vi "AMZ_S3_AUTH_Create Date Header String in UTC.vi"(8 "error in (no error)":errorcluster) -> (0 "error out":errorcluster, 3 "DateTime String (UTC)":string)   [LabVIEW 2015, in "LV Interface for Amazon S3.lvlib"]
doc: "Create the DateTime string in the format Amazon needs. This string is necessary for every request as the Date header's value."
uses:
  LV Interface for Amazon S3.lvlib
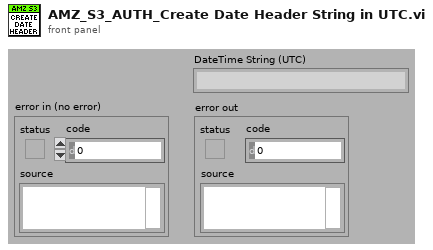
[diagram p1: front panel]
types:
  T1 = typedef "LVDateTimeRec.ctl" = cluster{"fractional second":dbl, "second":i32, "minute":i32, "hour":i32, "day of month":i32, "month":i32, "year":i32, "day of week":i32, "day of year":i32, "DST":i32}
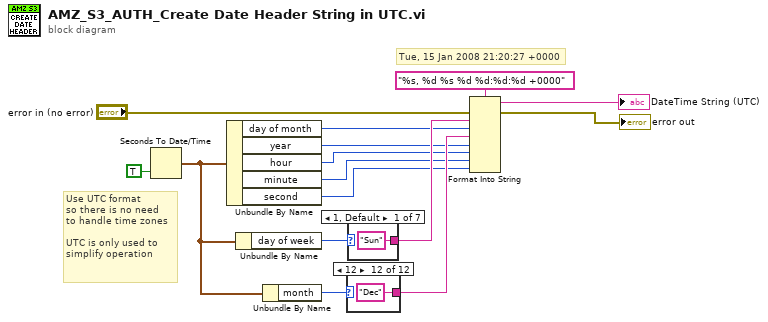
[diagram p0: block diagram]
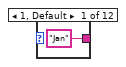
[diagram p2: hidden frame]
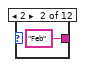
[diagram p3: hidden frame]
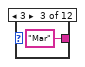
[diagram p4: hidden frame]
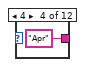
[diagram p5: hidden frame]
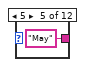
[diagram p6: hidden frame]
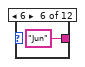
[diagram p7: hidden frame]
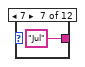
[diagram p8: hidden frame]
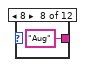
[diagram p9: hidden frame]
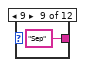
[diagram p10: hidden frame]
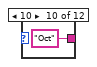
[diagram p11: hidden frame]
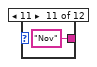
[diagram p12: hidden frame]
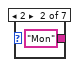
[diagram p13: hidden frame]
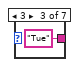
[diagram p14: hidden frame]
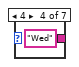
[diagram p15: hidden frame]
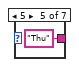
[diagram p16: hidden frame]
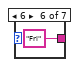
[diagram p17: hidden frame]
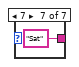
[diagram p18: hidden frame]
diagram:
  # "Use UTC format\nso there is no need\nto handle time zones\n\nUTC is only used to\nsimplify operation"
  # "Tue, 15 Jan 2008 21:20:27 +0000"
  n1 = Seconds To Date/Time(to UTC (F)=TRUE) -> (date time rec=w13:T1)  [unwired: 1 in]
  n2 = Unbundle By Name(w13) -> ("day of month"=w8:i32, "year"=w7:i32, "hour"=w6:i32, "minute"=w5:i32, "second"=w4:i32)
  n3 = Unbundle By Name(w13) -> ("day of week"=w14:i32)
  n4 = Unbundle By Name(w13) -> ("month"=w12:i32)
  n5 = case shown="12" w12 {
    tunnel: ["Jan" "Feb" "Mar" "Apr" "May" "Jun" "Jul" "Aug" "Sep" "Oct" "Nov" "Dec"] -> w9
    frame 1, Default {
    }
    frame 2 {
    }
    frame 3 {
    }
    frame 4 {
    }
    frame 5 {
    }
    frame 6 {
    }
    frame 7 {
    }
    frame 8 {
    }
    frame 9 {
    }
    frame 10 {
    }
    frame 11 {
    }
    frame 12 {
    }
  }
  n6 = case shown="1, Default" w14 {
    tunnel: ["Sun" "Mon" "Tue" "Wed" "Thu" "Fri" "Sat"] -> w10
    frame 1, Default {
    }
    frame 2 {
    }
    frame 3 {
    }
    frame 4 {
    }
    frame 5 {
    }
    frame 6 {
    }
    frame 7 {
    }
  }
  n7 = Format Into String(format string="%s, %d %s %d %d:%d:%d +0000", error in="error in (no error)", w10, w8, w9, w7, w6, w5, w4) -> (resulting string=→"DateTime String (UTC)":string, error out=→"error out":errorcluster)  [unwired: 1 in]
